vi "Read Dummy.vi"(8 "error in (no error)":errorcluster, 11 "Instance Handle":T1) -> (0 "error out":errorcluster, 2 "Dummy":bool, 3 "Session Handle":T1)   [LabVIEW 2020, in "singleton.lvclass"]
uses:
  singleton.lvclass
  Typedefs/Instance Handle.ctl
  singleton.lvclass/singleton.ctl
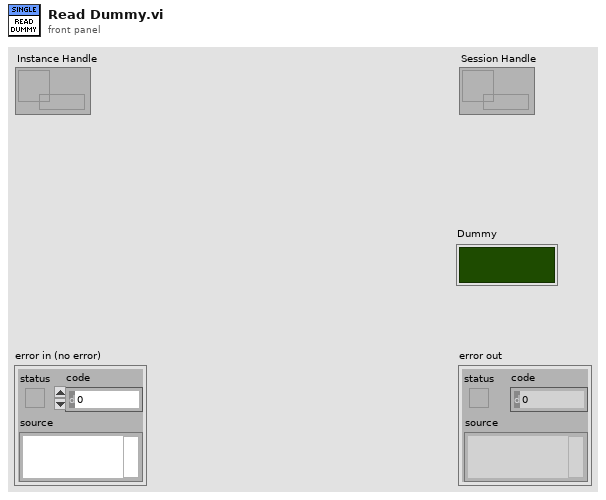
[diagram p1: front panel]
types:
  T1 = typedef "singleton.lvclass/Instance Handle.ctl" = refnum<data-value>
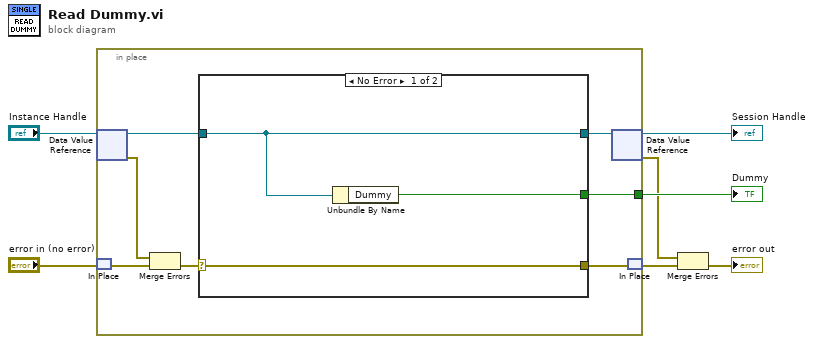
[diagram p0: block diagram]
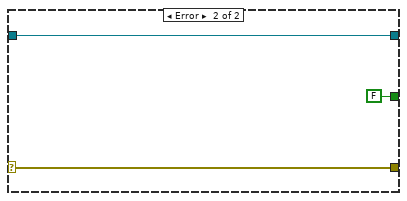
[diagram p2: hidden frame]
diagram:
  n1 = in-place {
    in-place-border: [w14] -> w7
    n2 = in-place-dvr #1("Instance Handle") -> (w9:refnum<class "singleton.lvclass">, w11:errorcluster)
    n3 = in-place-match #2("error in (no error)") -> (w13:errorcluster)
    n4 = Merge Errors(w11, w13) -> (w12:errorcluster)
    n5 = case shown="No Error" w12 {
      selector: w12 -> [w17 w20]
      tunnel: [w17 w20] -> w10
      tunnel: [w16 FALSE ("Dummy")] -> w14
      tunnel: w9 -> [w15 w19]
      tunnel: [w15 w19] -> w8
      frame No Error {
        n6 = Unbundle By Name(w15) -> ("Dummy"=w16:bool)
      }
      frame Error {
      }
    }
    n7 = in-place-dvr #1(w8) -> (→"Session Handle":T1, w4:errorcluster)
    n8 = in-place-match #2(w10) -> (w5:errorcluster)
  }
  "Dummy" <- w7
  n9 = Merge Errors(w4, w5) -> (→"error out":errorcluster)
